vi "HTTP_GET_EXAMPLE.vi"() -> ()   [LabVIEW 2018]
uses:
  <vilib>/httpClient/LabVIEWHTTPClient.lvlib
panel:
  out "body":string
  out "headers":string
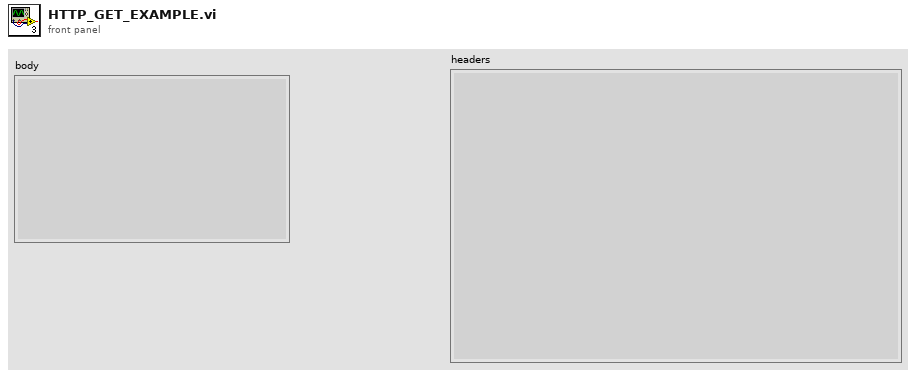
[diagram p1: front panel]
types:
  T1 = typedef "LabVIEWHTTPClient.lvlib/ClientHandle.ctl" = refnum<k1>
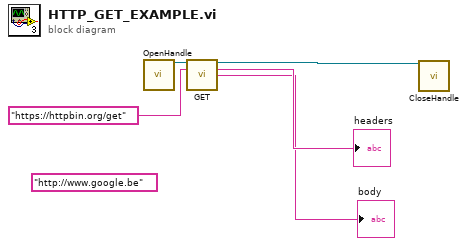
[diagram p0: block diagram]
diagram:
  (unwired) "http://www.google.be" ("url")
  n1 = call <vilib>:"OpenHandle.vi"() -> ("client handle out"=w5:T1)  [unwired: 14 in, 1 out]
  n2 = call <vilib>:"GET.vi"("client handle"=w5, "url"="https://httpbin.org/get") -> ("client handle out"=w4:T1, "headers"=→"headers":string, "body"=→"body":string)  [unwired: 10 in, 1 out]
  n3 = call <vilib>:"CloseHandle.vi"("client handle"=w4) -> ()  [unwired: 14 in, 1 out]
